vi "ECOG-Initialize Display.vi"(0 "params":T2, 7 "ref":refnum<vi>, 11 "error in (no error)":errorcluster) -> (4 "params thru":T2, 13 "display":T1 {"IIR Filter"."Forward Coefficients" format="%.4f"; "IIR Filter"."Reverse Coefficients" format="%.4f"}, 15 "error out":errorcluster)   [LabVIEW 2020]
uses:
  Typedefs/ECOG-Parameters.ctl
  Typedefs/ECOG-Display.ctl
  <vilib>/Analysis/3filter.llb/Filter Passband Type.ctl
  epl-vi-lib/Utility VIs/Math VIs/LinSpace (x0-dx-npts).vi
  <vilib>/Analysis/NI_AALBase.lvlib
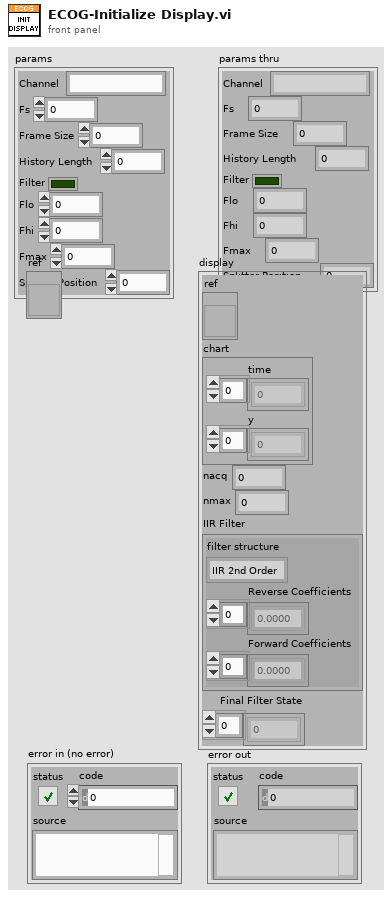
[diagram p1: front panel]
types:
  T1 = typedef "ECOG-Display.ctl" = cluster{"ref":refnum<vi>, "chart":cluster{"time":dbl[], "y":dbl[]}, "nacq":i32, "nmax":i32, "IIR Filter":cluster{"filter structure":enum32{"IIR 2nd Order", "IIR 4th Order"}, "Reverse Coefficients":dbl[], "Forward Coefficients":dbl[]}, "Final Filter State":dbl[]}
  T2 = typedef "ECOG-Parameters.ctl" = cluster{"Channel":string, "Fs":dbl, "Frame Size":dbl, "History Length":dbl, "Filter":bool, "Flo":dbl, "Fhi":dbl, "Fmax":dbl, "Splitter Position":i32}
  T3 = typedef "NI_AALBase.lvlib/Filter Passband Type.ctl" = enum32{"Lowpass", "Highpass", "Bandpass", "Bandstop"}
  T4 = cluster{"filter structure":enum32{"IIR 2nd Order", "IIR 4th Order"}, "Reverse Coefficients":dbl[], "Forward Coefficients":dbl[]}
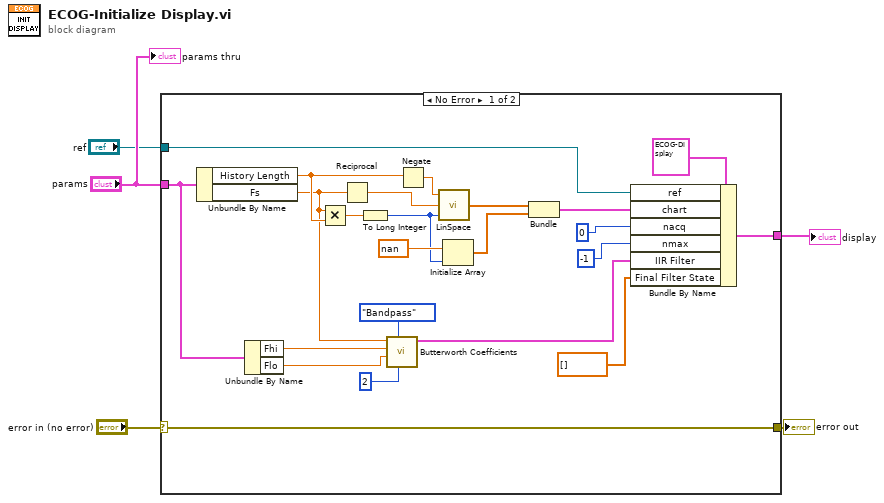
[diagram p0: block diagram]
diagram:
  n1 = case shown="No Error" "error in (no error)" {
    selector: "error in (no error)" -> [w19 w29]
    tunnel: "params" -> [w11 _]
    tunnel: [w19 w29] -> w4
    tunnel: "ref" -> [w22 _]
    tunnel: [w20 _] -> w1
    frame No Error {
      n2 = Unbundle By Name(w11) -> ("History Length"=w17:dbl, "Fs"=w12:dbl)
      n3 = Unbundle By Name(w11) -> ("Fhi"=w10:dbl, "Flo"=w9:dbl)
      n4 = Multiply(x=w12, y=w17) -> (x*y=w28:dbl)
      n5 = Reciprocal(x=w12) -> (1/x=w23:dbl)
      n6 = To Long Integer(number=w28) -> (32bit integer=w25:i32)
      n7 = call <vilib>:"Butterworth Coefficients.vi"("order"=2, "filter type"=Filter_Passband_Type."Bandpass", "low cutoff freq: fl"=w9, "high cutoff freq: fh"=w10, "sampling freq: fs"=w12) -> ("IIR Filter Cluster"=w7:T4)  [unwired: 5 in, 1 out]
      n8 = Negate(x=w17) -> (-x=w18:dbl)
      n9 = call-poly "LinSpace.vi"("npts"=w25, "dx"=w23, "x0"=w18) -> ("Array"=w24:dbl[])  [unwired: 1 in, 1 out]
      n10 = Initialize Array(nan, w25) -> (w26:dbl[])
      n11 = Bundle("Array"=w24, w26) -> (w21:cluster{"Array":dbl[], dbl[]})  [unwired: 1 in]
      n12 = Bundle By Name(cluster=T1 {"ref"=refnum, "chart"={"time"=[], "y"=[]}, "nacq"=0, "nmax"=0, "IIR Filter"={"filter structure"=enum."IIR 2nd Order", "Reverse Coefficients"=[], "Forward Coefficients"=[]}, "Final Filter State"=[]} ("display"), "ref"=w22, "chart"=w21, "nacq"=0, "nmax"=-1, "IIR Filter"=w7, "Final Filter State"=dbl[] []) -> (w20:T1)
    }
    frame Error {
    }
  }
  "error out" <- w4
  "display" <- w1
  "params thru" <- "params"
